vi "HEWH Calculate Cp Water.vi"(11 "RTD Out (Deg F)":dbl) -> (3 "Cp Water":dbl)   [LabVIEW 2016]
uses:
  <vilib>/Analysis/6fits.llb/Curve Fitting Criteria.ctl
  <vilib>/Analysis/6fits.llb/General Linear Fit Algorithm.ctl
  <vilib>/Analysis/NI_AALPro.lvlib
panel:
  out "Best Polynomial Fit":dbl[](array[numeric])
  out "Polynomial Coefficients":dbl[](array[numeric])
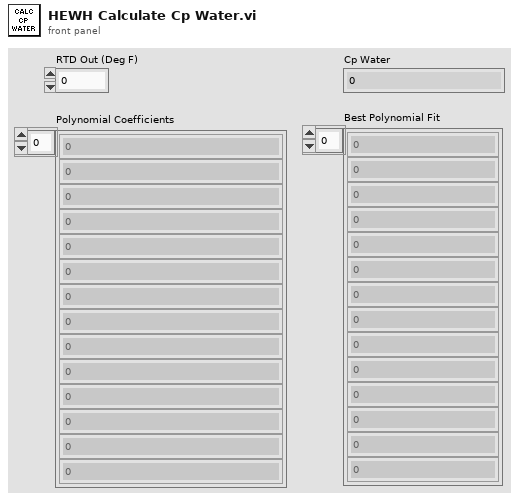
[diagram p1: front panel]
types:
  T1 = typedef "NI_AALPro.lvlib/General Linear Fit Algorithm.ctl" = u16
  T2 = typedef "NI_AALPro.lvlib/Curve Fitting Criteria.ctl" = u16
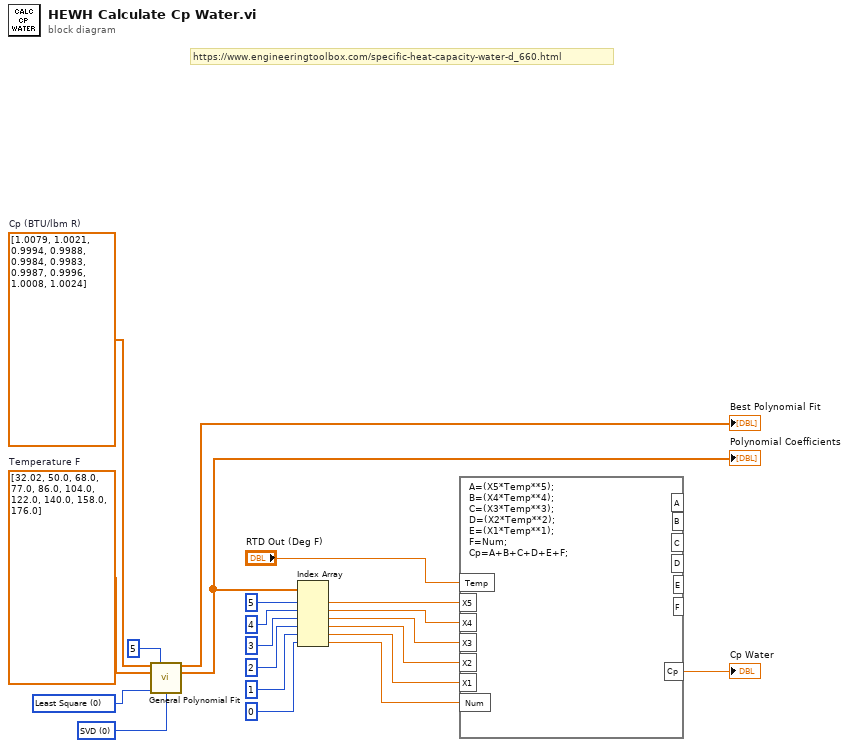
[diagram p0: block diagram]
diagram:
  w3 = T1 0 items=["SVD", "Givens", "Givens2", "Householder", "LU Decomposition", "Cholesky", "SVD for Rank Deficient H"] ("algorithm")
  w19 = T2 0 items=["Least Square", "Least Absolute Residual", "Bisquare"] ("method")
  w20 = dbl[] [1.0079, 1.0021, 0.9994, 0.9988, 0.9984, 0.9983, 0.9987, 0.9996, 1.0008, 1.0024]  # Cp (BTU/lbm R)
  w21 = dbl[] [32.02, 50.0, 68.0, 77.0, 86.0, 104.0, 122.0, 140.0, 158.0, 176.0]  # Temperature F
  # "https://www.engineeringtoolbox.com/specific-heat-capacity-water-d_660.html"
  n1 = call <vilib>:"General Polynomial Fit.vi"("Y"=w20, "polynomial order"=5, "X"=w21, "method"=w19, "algorithm"=w3) -> ("Best Polynomial Fit"=→"Best Polynomial Fit":dbl[], "Polynomial Coefficients"=w2:dbl[])  [unwired: 7 in, 2 out]
  "Polynomial Coefficients" <- w2
  n2 = Index Array(array=w2, index #1=5 ("index"), index #2=4 ("index"), index #3=3 ("index"), index #4=2 ("index"), index #5=1 ("index"), index #6=0 ("index")) -> (element #1=w11:dbl, element #2=w10:dbl, element #3=w9:dbl, element #4=w8:dbl, element #5=w4:dbl, element #6=w7:dbl)
  n3 = formula code="A=(X5*Temp**5);\nB=(X4*Temp**4);\nC=(X3*Temp**3);\nD=(X2*Temp**2);\nE=(X1*Temp**1);\nF=Num;\nCp=A+B+C+D+E+F;"("X5"=w11, "X4"=w10, "X3"=w9, "X2"=w8, "X1"=w4, "Num"=w7, "Temp"="RTD Out (Deg F)") -> ("Cp"=→"Cp Water":dbl)  [unwired: 6 out]
